vi "Get Incorrect IPG Temp Cal Information.vi"(8 "error in":errorcluster, 11 "Manifold Ambient Temperature":dbl=nan) -> (0 "error out":errorcluster, 1 "Incorrect IPG Reported Temperature (42C)":dbl=nan, 2 "Incorrect IPG Reported Temperature (41C)":dbl=nan, 3 "Incorrect IPG Reported Temperature (40C)":dbl=nan, 4 "Gen Cals":string, 5 "Incorrect IPG Reported Temperature (10C)":dbl=nan)   [LabVIEW 2010]
doc: "This function sends a Telemetry query to the IPG for General Calibration status including Temperature Thresholds (ohms). The Temperature Thresholds are converted from ohms to degrees Celsius.\n\nIf the status string format is incorrect, <not available> and NaN values will be returned."
uses:
  Drivers/Telemetry/Typedef Command List.ctl
panel:
  out "Initial Offset Ratio (42C)":dbl=nan
  out "Initial Offset Ratio (41C)":dbl=nan
  out "Initial Offset Ratio (40C)":dbl=nan
  out "Initial Offset Ratio (10C)":dbl=nan
  in  "Ideal Abort Threshold (R @ 42C)":dbl=46875.0
  in  "Ideal Critical Threshold (R @ 41C)":dbl=48917.0
  in  "Ideal Warning Threshold (R @ 40C)":dbl=51060.0
  in  "Ideal Minimum Threshold (R @ 10C)":dbl=207801.0
  out "Abort Threshold (ohms)":dbl=nan format="%.1f"
  out "Critical Threshold (ohms)":dbl=nan format="%.1f"
  out "Warning Threshold (ohms)":dbl=nan format="%.1f"
  out "Min Threshold (ohms)":dbl=nan format="%.1f"
  # "Get General Calibration\nfrom IPG"
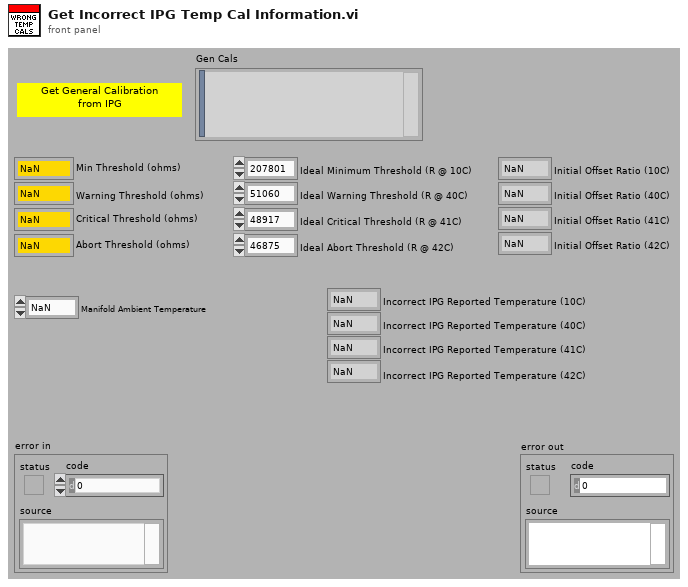
[diagram p1: front panel]
types:
  T1 = typedef "Typedef Command List.ctl" = enum16{"Get xPG Status", "xPG Stimulation", "Select Program", "Increment Program Amplitude", "Decrement Program Amplitude", "Get PoP Constants", "Get PPC Constants", "Get Program Names", "Set Pulse Amplitude", "Increment Pulse Amplitude", "Decrement Pulse Amplitude", "Get Pulse Widths", "Set Pulse Widths", "Increment Pulse Width", "Decrement Pulse Width", "Get Program Frequency", "Set Program Frequency", "Increment Program Frequency", "Decrement Program Frequency", "Inject Event", "Charging Control", "Get xPG Identity", "Set xPG Identity", "Restore Program Defaults", "Get Program Definition", "Set Program Definition", "Get Program Constants", "Set Program Constants", "Get Configurable Device Parameters", "Set Configurable Device Parameters", "Get Pulse Constants", "Set Pulse Constants", "Get Lead Limits", "Set Lead Limits", "Get Channel Calibrations", "Set Channel Calibrations", "<reserved 2>", "<reserved 3>", "<reserved 4>", "<reserved 5>", "<reserved 6>", "<reserved 7>", "Get Stim Asic HV Calibrations", "Set Stim Asic HV Calibrations", "<reserved 8>", "<reserved 9>", "Get CP Data", "Set CP Data", "Clear Log", "Read Log", "Append Log", "Get Patient Program Runtime", "Set Patient Program Runtime", "Impedance Measurement", "Enter Storage Mode", "Echo Short", "Echo Long", "Get General Calibration", "Set General Calibration", "Get Trim List", "Set Trim List", "Get Counter", "Set Counter", "Get Test Stimulation", "Set Test Stimulation", "Get Titration Stimulation", "Set Titration Stimulation", "Get Ramp Time", "Set Ramp Time", "Get VBAT", "Set Software Description Block", "Get Software Description Block", "Write Memory", "Read Memory", "Reset xPG", "Erase Flash Block", "Write Vectors", "Read Vectors", "Diagnostic Data", "Set Background Impedance", "Get Background Impedence ", "Set Test Waveform", "Calibrate Channel", "Get Log Range", "Reserved 0x55", "Reserved 0x56", "MICS Options", "Pair PPC", "Pair POP", "Stop Bootloader", "Tune MICS", "MICS Diagnostics", "Undefined"}
  T2 = cluster{"Command":T1, "Function":enum16{"Open Session", "Close Session", "Downlink Only", "Uplink Only", "Transceive (DN -> UP)"}, "MICS_ID":u32, "EXID":u32, "Use Local":bool, "Transceive Delay mS":dbl, "CP_DATA IN":u8[], "Parameters":string}
  T3 = enum16{"Open Session", "Close Session", "Downlink Only", "Uplink Only", "Transceive (DN -> UP)"}
  T4 = cluster{"Response Token":string, "Response Code":string, "bChecksum Valid":bool, "tChecksum Valid":bool, "CP_DATA OUT":u8[], "Data":string}
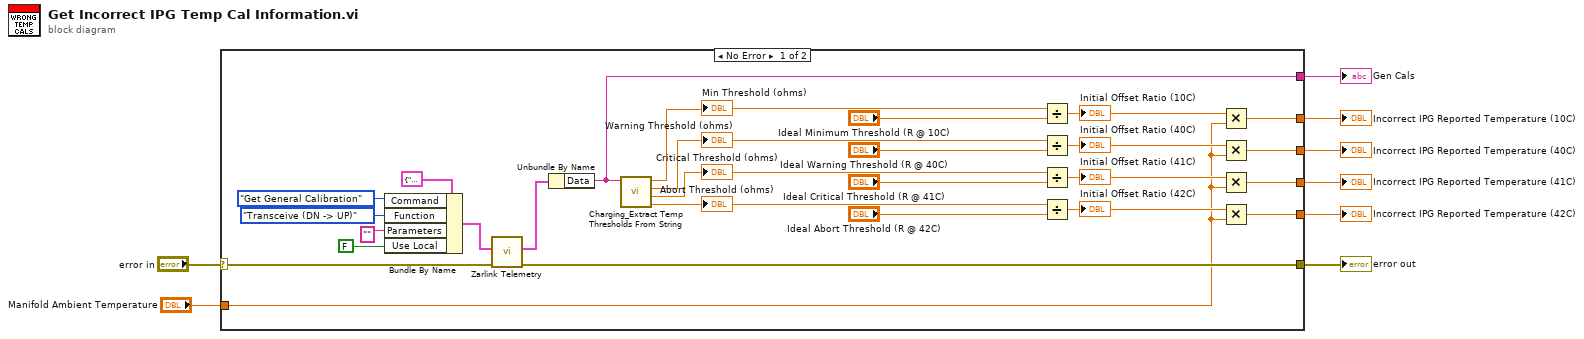
[diagram p0: block diagram]
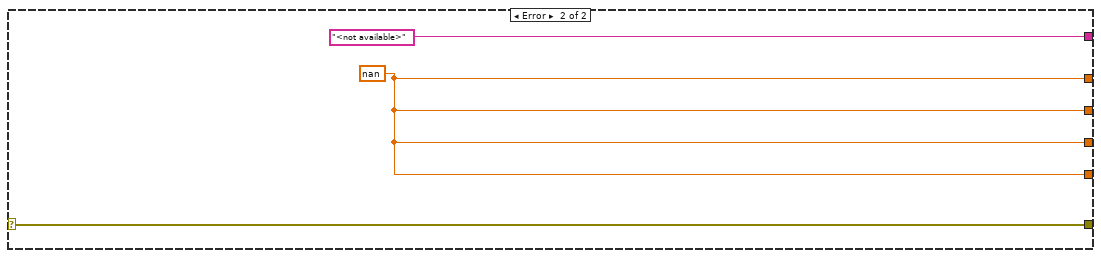
[diagram p2: hidden frame]
diagram:
  n1 = case shown="No Error" "error in" {
    selector: "error in" -> [w27 w36]
    tunnel: [w35 w36] -> w8
    tunnel: [w17 w37] -> w5
    tunnel: [w16 w37] -> w4
    tunnel: [w15 w37] -> w3
    tunnel: [w14 w37] -> w2
    tunnel: [w26 "<not available>" ("Data")] -> w6
    tunnel: "Manifold Ambient Temperature" -> [w13 _]
    frame No Error {
      n2 = Bundle By Name(cluster=T2 {"Command"=enum."Get xPG Status", "Function"=enum."Close Session", "MICS_ID"=0, "EXID"=16773121, "Use Local"=FALSE, "Transceive Delay mS"=100.0, "CP_DATA IN"=[], "Parameters"=""} ("Input"), "Command"=Typedef_Command_List."Get General Calibration", "Function"=T3."Transceive (DN -> UP)", "Parameters"="", "Use Local"=FALSE) -> (w34:T2)
      n3 = call "Zarlink Telemetry.vi"("error in (no error)"=w27, "Input"=w34) -> ("error out"=w35:errorcluster, "Output"=w30:T4)  [unwired: 7 in, 1 out]
      n4 = Unbundle By Name(w30) -> ("Data"=w26:string)
      n5 = call "Charging_Extract Temp Thresholds From String.vi"("Gen Cals In"=w26) -> ("Abort Thresholdl (ohms)"=w12:dbl, "Critical Thresholdl (ohms)"=w11:dbl, "Warning Thresholdl (ohms)"=w10:dbl, "Min Threshold (ohms)"=w9:dbl)  [unwired: 7 in]
      "Min Threshold (ohms)" <- w9
      "Warning Threshold (ohms)" <- w10
      "Critical Threshold (ohms)" <- w11
      "Abort Threshold (ohms)" <- w12
      n6 = Divide(x=w9, y="Ideal Minimum Threshold (R @ 10C)") -> (x/y=w21:dbl)
      "Initial Offset Ratio (10C)" <- w21
      n7 = Divide(x=w10, y="Ideal Warning Threshold (R @ 40C)") -> (x/y=w20:dbl)
      "Initial Offset Ratio (40C)" <- w20
      n8 = Divide(x=w11, y="Ideal Critical Threshold (R @ 41C)") -> (x/y=w19:dbl)
      "Initial Offset Ratio (41C)" <- w19
      n9 = Divide(x=w12, y="Ideal Abort Threshold (R @ 42C)") -> (x/y=w18:dbl)
      "Initial Offset Ratio (42C)" <- w18
      n10 = Multiply(x=w21, y=w13) -> (x*y=w17:dbl)
      n11 = Multiply(x=w20, y=w13) -> (x*y=w16:dbl)
      n12 = Multiply(x=w19, y=w13) -> (x*y=w15:dbl)
      n13 = Multiply(x=w18, y=w13) -> (x*y=w14:dbl)
    }
    frame Error {
      w37 = nan ("tempWarningThresholdl (ohms)")
    }
  }
  "error out" <- w8
  "Gen Cals" <- w6
  "Incorrect IPG Reported Temperature (10C)" <- w5
  "Incorrect IPG Reported Temperature (40C)" <- w4
  "Incorrect IPG Reported Temperature (41C)" <- w3
  "Incorrect IPG Reported Temperature (42C)" <- w2
